vi "Renishaw-XL80_Close.vi"(8 "error in (no error)":errorcluster, 11 "Renishaw-XL80 in":refnum<class "Renishaw-XL80.lvclass">) -> (0 "error out":errorcluster, 3 "Renishaw-XL80 out":refnum<class "Renishaw-XL80.lvclass">)   [LabVIEW 2024, in "Renishaw-XL80.lvclass"]
doc: "This method disconnects a client from a DX10.\n\nDefinition\nHRESULTDisconnect();\nParameters\nNone\n\n\nComments\nThis method must be called before the client exits. Failing to call this method will at best lead to a reference leak and at worst can mean that the DX10 remains unavailable to other clients.\n\nA similar effect may occur if the client crashes before calling this method. In both cases restarting DX10Server.exe is the only way to recover.\n\nThis method will normally return with an HRESULT of S_OK unless there is an unexpected error. \n\nSee Also"
uses:
  Renishaw-XL80.lvclass
  Renishaw-XL80.lvclass/Renishaw-XL80.ctl
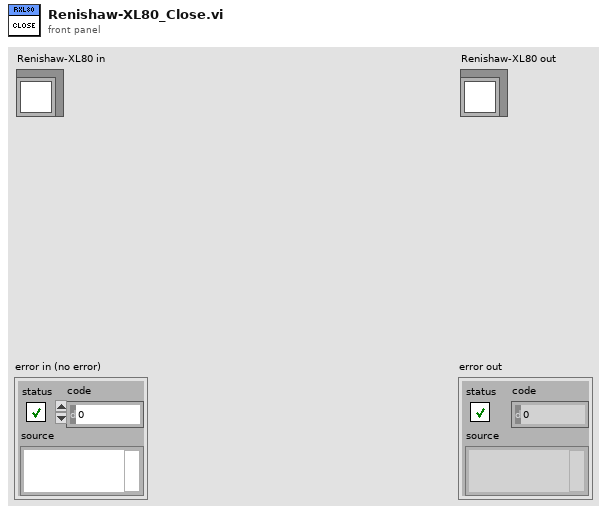
[diagram p1: front panel]
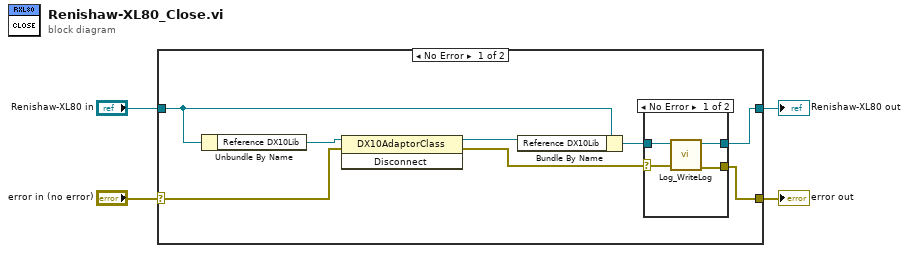
[diagram p0: block diagram]
diagram:
  n1 = case shown="No Error" "error in (no error)" {
    selector: "error in (no error)" -> [w9 w20]
    tunnel: [w5 w20] -> w3
    tunnel: [w7 w19] -> w1
    tunnel: "Renishaw-XL80 in" -> [w10 w19]
    frame No Error {
      n2 = Unbundle By Name(w10) -> ("Reference DX10Lib"=w12:refnum<k24>)
      n3 = invoke class="DX10AdaptorClass" method="Disconnect"(reference=w12, error in=w9) -> (reference out=w11:refnum<k24>, error out=w6:errorcluster)  [unwired: 1 in, 1 out]
      n4 = Bundle By Name(cluster=w10, "Reference DX10Lib"=w11) -> (w8:refnum<class "Renishaw-XL80.lvclass">)
      n5 = case shown="No Error" w6 {
        selector: w6 -> [w14 w17]
        tunnel: w8 -> [w16 w18]
        tunnel: [w15 w18] -> w7
        tunnel: [w13 w17] -> w5
        frame No Error {
          n6 = call-dynamic "Log_WriteLog.vi"("error in (no error)"=w14, "Log in"=w16) -> ("error out"=w13:errorcluster, "Log out"=w15:refnum<class "Renishaw-XL80.lvclass">)  [unwired: 8 in]
        }
        frame Error {
        }
      }
    }
    frame Error {
    }
  }
  "error out" <- w3
  "Renishaw-XL80 out" <- w1
